vi "loop-timer.vi"(11 "loop-time-in":u32) -> (1 "Loop Time (mS)":u32, 3 "loop-time-out":u32, 4 "Hz":dbl)   [LabVIEW 2020]
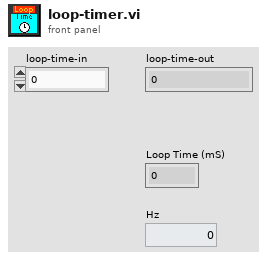
[diagram p1: front panel]
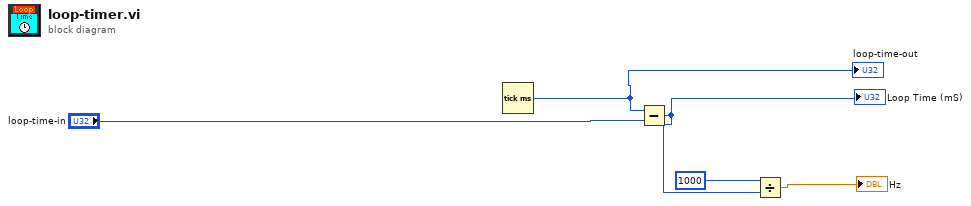
[diagram p0: block diagram]
diagram:
  n1 = Tick Count (ms)() -> (millisecond timer value=w4:u32)
  "loop-time-out" <- w4
  n2 = Subtract(x=w4, y="loop-time-in") -> (x-y=w2:u32)
  "Loop Time (mS)" <- w2
  n3 = Divide(x=u32 1000 ("y"), y=w2) -> (x/y=→"Hz":dbl)
